vi "Consulter_Bilan.vi"() -> ()   [LabVIEW 2024]
uses:
  SurveillancePanel/CustomizedAssets/text_indicator.ctl
panel:
  out "Image":T1(plugin-control)
  out "Localisation":string
  out "Date":string
  out "Nombre de \nvéhicules suspects:":dbl
  out "Nombre de véhicules:":dbl
  in  "Consulter Bilan":bool
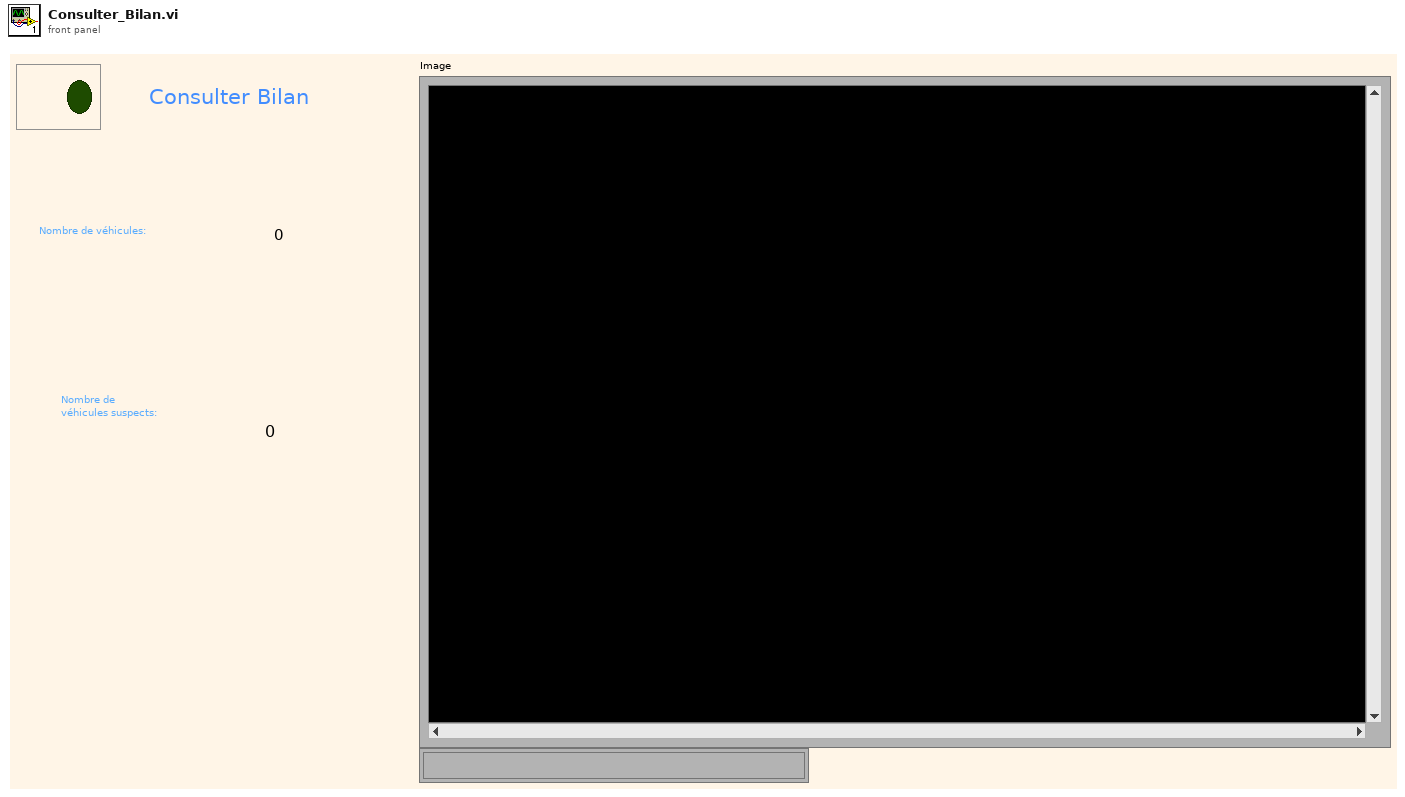
[diagram p1: front panel]
types:
  T1 = typedef "IMAQ Image.ctl" = refnum<image>
  T2 = typedef "text_indicator.ctl" = string
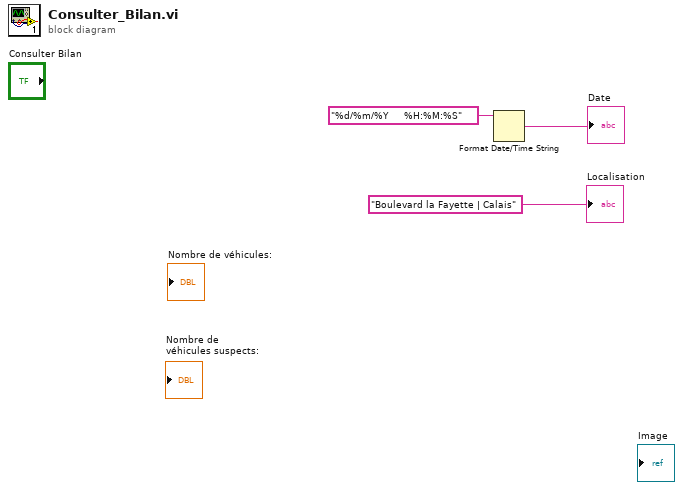
[diagram p0: block diagram]
diagram:
  n1 = Format Date/Time String(time format string (%c)="%d/%m/%Y     %H:%M:%S") -> (date/time string=→"Date":string)  [unwired: 2 in]
  "Localisation" <- T2 "Boulevard la Fayette | Calais" ("Localisation")
